vi "Module - RH_JENGENG.vi"() -> ()   [LabVIEW 2019]
uses:
  Control/State - eFGV.ctl
panel:
  out "Site Name":string="RH BELAJA (22.75 kWp)"
  out "STP-03-B-IDC":dbl caption="B.Idc" format="%.1f A"
  out "STP-03-B-VDC":dbl caption="B.Vdc" format="%.0f V"
  out "STP-02-B-IDC":dbl caption="B.Idc" format="%.1f A"
  out "STP-02-B-VDC":dbl caption="B.Vdc" format="%.0f V"
  out "STP-01-B-IDC":dbl caption="B.Idc" format="%.1f A"
  out "STP-01-B-VDC":dbl caption="B.Vdc" format="%.0f V"
  out "BANK-04-STATUS":bool
  out "BANK-03-STATUS":bool
  out "BANK-02-STATUS":bool
  out "BANK-01-STATUS":bool
  out "BANK-04-TEMP":dbl caption="T_bat" format="%#_g °C"
  out "BANK-04-IDC":dbl caption="I_bat" format="%.2f A"
  out "BANK-04-VDC":dbl caption="V_bat" format="%.1f V"
  out "BANK-04-SOC":dbl caption="SOC" format="%#_g %"
  out "BANK-03-TEMP":dbl caption="T_bat" format="%#_g °C"
  out "BANK-03-IDC":dbl caption="I_bat" format="%.2f A"
  out "BANK-03-VDC":dbl caption="V_bat" format="%.1f V"
  out "BANK-03-SOC":dbl caption="SOC" format="%#_g %"
  out "SI-M-02-STATUS":bool
  out "SI-M-02-FREQ":dbl caption="FREQ" format="%.0f Hz"
  out "SI-M-02-L3":dbl caption="L3" format="%.0f V"
  out "SI-M-02-L2":dbl caption="L2" format="%.0f V"
  out "SI-M-02-L1":dbl caption="L1" format="%.0f V"
  out "SI-M-02-PAC":dbl caption="Pac" format="%.0f W"
  out "STP-03-STATUS":bool
  out "STP-03-A-IDC":dbl caption="A.Idc" format="%.1f A"
  out "STP-03-A-VDC":dbl caption="A.Vdc" format="%.0f V"
  out "STP-03-PAC":dbl caption="Pac" format="%#_g W"
  out "PM-01-STATUS":bool
  out "SI-M-01-STATUS":bool
  out "STP-02-STATUS":bool
  out "STP-01-STATUS":bool
  out "BANK-02-TEMP":dbl caption="T_bat" format="%#_g °C"
  out "BANK-02-IDC":dbl caption="I_bat" format="%.2f A"
  out "BANK-02-VDC":dbl caption="V_bat" format="%.1f V"
  out "BANK-02-SOC":dbl caption="SOC" format="%#_g %"
  out "STP-02-A-IDC":dbl caption="A.Idc" format="%.1f A"
  out "STP-02-A-VDC":dbl caption="A.Vdc" format="%.0f V"
  out "STP-02-PAC":dbl caption="Pac" format="%#_g W"
  out "PM-01-FREQ":dbl caption="Freq" format="%.0f Hz"
  out "PM-01-IAC":dbl caption="Iac" format="%.0f A"
  out "PM-01-VAC":dbl caption="Vac" format="%.0f V"
  out "PM-01-PAC":dbl caption="Pac" format="%.0f W"
  out "SI-M-01-FREQ":dbl caption="FREQ" format="%.0f Hz"
  out "SI-M-01-L3":dbl caption="L3" format="%.0f V"
  out "SI-M-01-L2":dbl caption="L2" format="%.0f V"
  out "SI-M-01-L1":dbl caption="L1" format="%.0f V"
  out "SI-M-01-PAC":dbl caption="Pac" format="%.0f W"
  out "BANK-01-TEMP":dbl caption="T_bat" format="%#_g °C"
  out "BANK-01-IDC":dbl caption="I_bat" format="%.2f A"
  out "BANK-01-VDC":dbl caption="V_bat" format="%.1f V"
  out "BANK-01-SOC":dbl caption="SOC" format="%#_g %"
  out "STP-01-A-IDC":dbl caption="A.Idc" format="%.1f A"
  out "STP-01-A-VDC":dbl caption="A.Vdc" format="%.0f V"
  out "STP-01-PAC":dbl caption="Pac" format="%.0f W"
  # "RH JENGENG (30.3 kWp)"
  # "BANK-1"
  # "BANK-2"
  # "BANK-1"
  # "BANK-2"
  # "STP-01"
  # "STP-02"
  # "SI-M-01"
  # "SI-M-02"
  # "STP-03"
  # "PM-01"
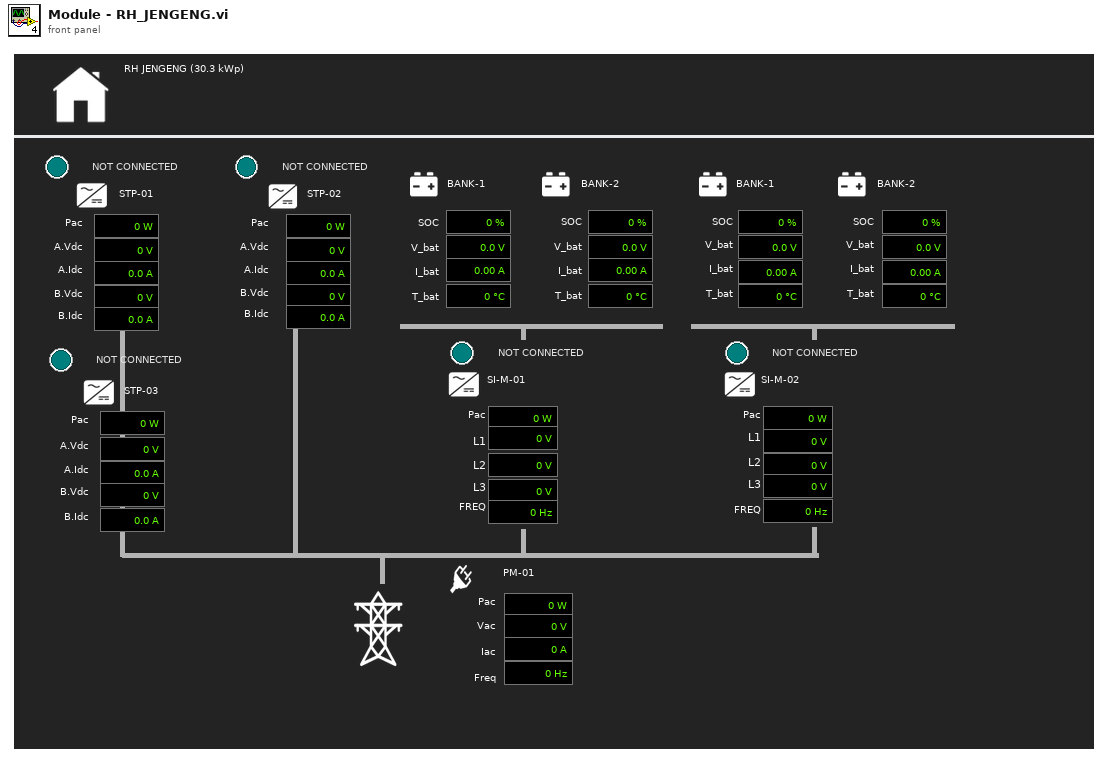
[diagram p1: front panel]
types:
  T1 = typedef "State - eFGV.ctl" = enum16{"Init", "Read", "Write", "Close"}
  T2 = typedef "Device Name.ctl" = enum16{"SB-01", "SB-02", "SB-03", "SB-04", "STP-01", "STP-02", "STP-03", "STP-04", "BANK-01", "BANK-02", "BANK-03", "BANK-04", "SI-M-01", "SI-M-02", "SI-M-03", "SI-M-04", "PM-01", "PM-02", "PM-03", "PM-04"}
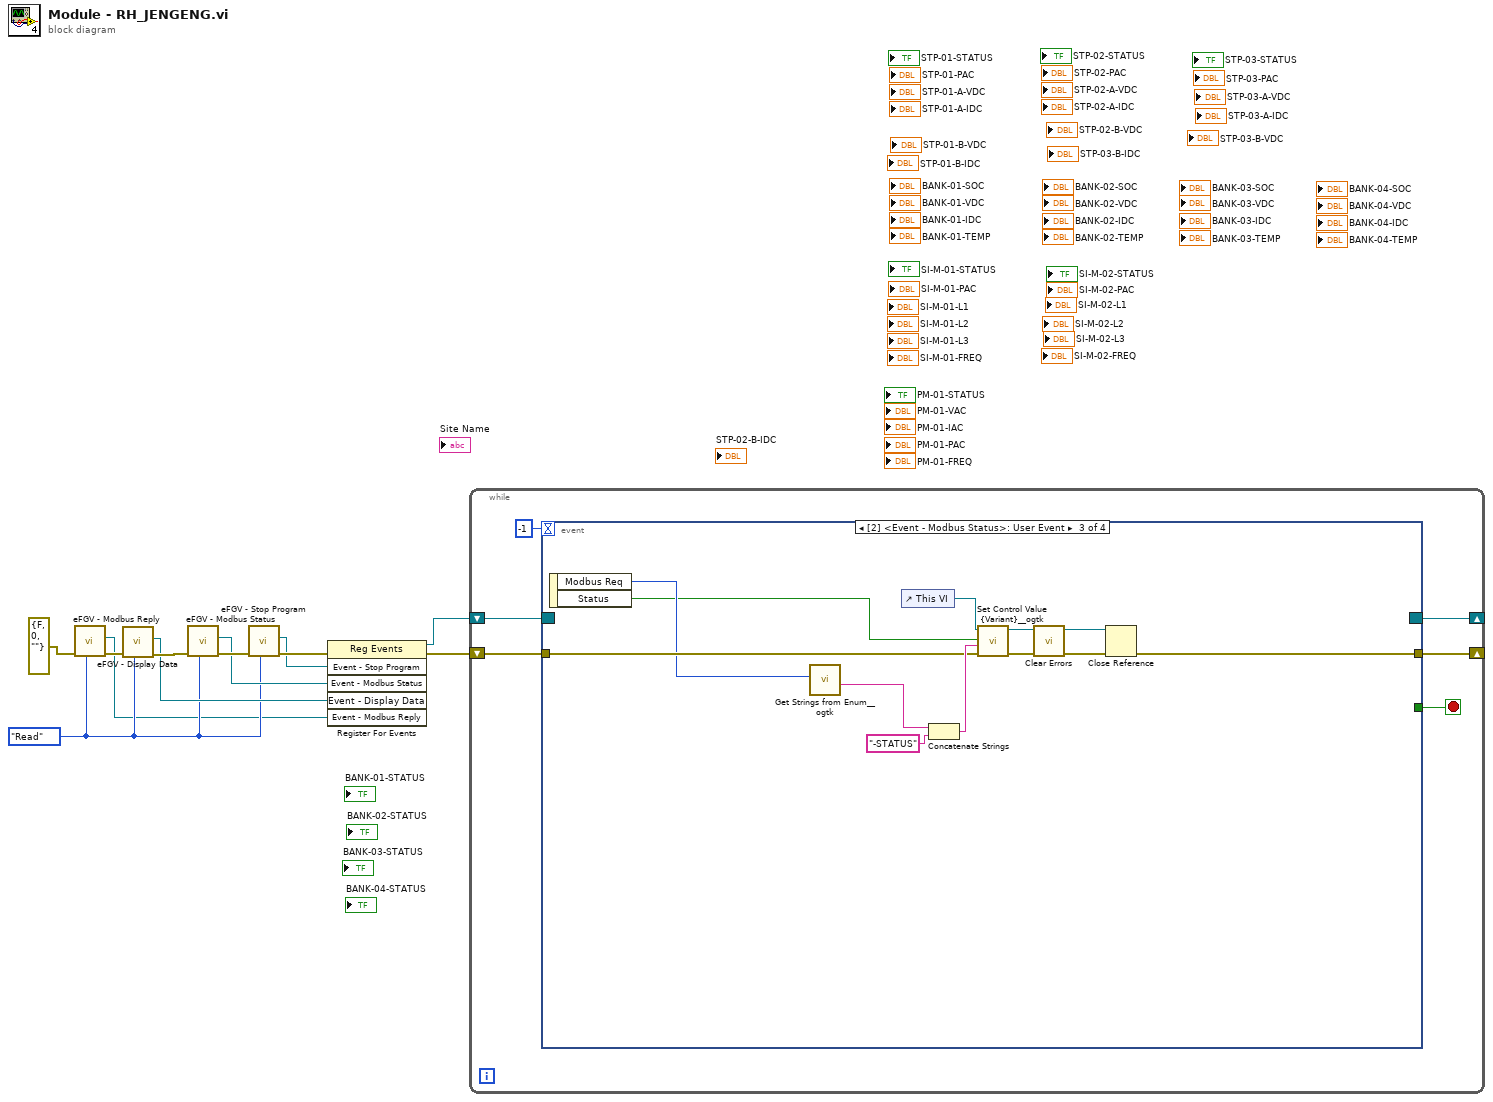
[diagram p0: block diagram]
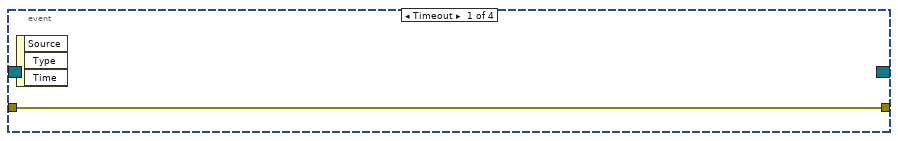
[diagram p2: hidden frame]
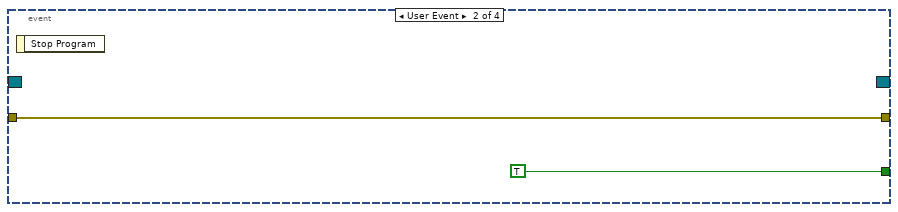
[diagram p3: hidden frame]
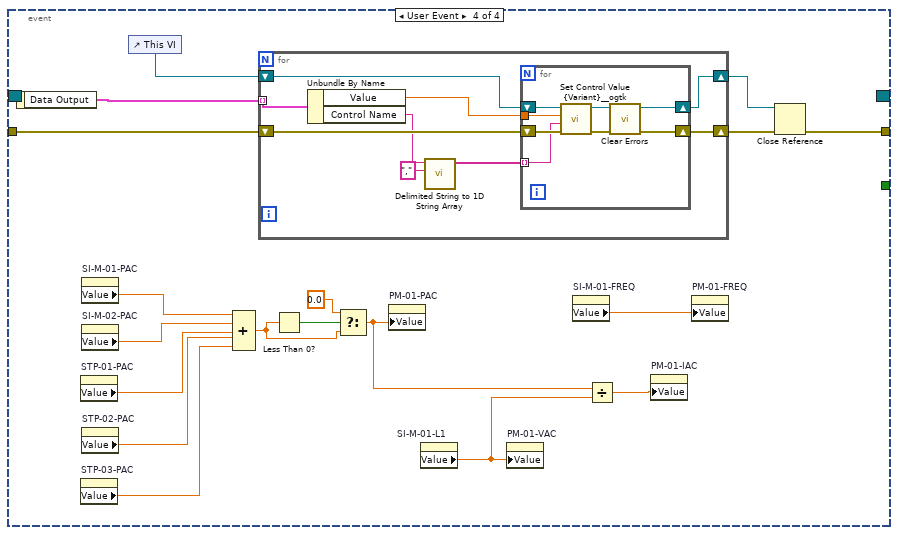
[diagram p4: hidden frame]
diagram:
  w2 = State_-_eFGV."Read" ("State - eFGV")
  n1 = call "eFGV - Modbus Reply.vi"("State - eFGV"=w2, "error in (no error)"=errorcluster {"status"=FALSE, "code"=0, "source"=""}) -> ("error out"=w3:errorcluster, "Event - Modbus Reply"=w1:refnum<user-event>)  [unwired: 8 in]
  n2 = call "eFGV - Display Data.vi"("State - eFGV"=w2, "error in (no error)"=w3) -> ("error out"=w7:errorcluster, "Event - Display Data"=w6:refnum<user-event>)  [unwired: 8 in]
  n3 = call "eFGV - Modbus Status.vi"("State - eFGV"=w2, "error in (no error)"=w7) -> ("error out"=w9:errorcluster, "Event - Modbus Status"=w8:refnum<user-event>)  [unwired: 8 in]
  n4 = call "eFGV - Stop Program.vi"("State - eFGV"=w2, "error in (no error)"=w9) -> ("error out"=w12:errorcluster, "Event - Stop Program"=w11:refnum<user-event>)  [unwired: 8 in]
  n5 = register-events(error in=w12, w11, w8, w6, w1) -> (reference out=w10:refnum<event-registration>, error out=w5:errorcluster)  [unwired: 1 in]
  n6 = while {
    shift-right: [w17] -> _
    shift-left: w10 -> [w18]
    shift-right: [w14] -> _
    shift-left: w5 -> [w13]
    stop <- w16 stop-if-true
    n7 = event shown="[2] <Event - Modbus Status>: User Event" {
      selector: w18 -> [_ _ _ _]
      dyn-events: [_ _ _ _] -> w17
      timeout: -1 -> [_ _ _ _]
      tunnel: w13 -> [w19 w20 w26 w46]
      tunnel: [_ TRUE _ _] -> w16
      tunnel: [w19 w20 w23 w48] -> w14
      event Timeout {
        n8 = event-data() -> ()  [unwired: 1 in, 3 out]
      }
      event User Event {
        n9 = event-data() -> ()  [unwired: 1 in, 1 out]
      }
      event User Event {
        n10 = event-data() -> ("Modbus Req"=w25:T2, "Status"=w24:bool)  [unwired: 1 in]
        n11 = call "Get Strings from Enum__ogtk.vi"("Enum"=w25) -> ("String Value"=w28:string)  [unwired: 7 in, 3 out]
        n12 = control-ref of="This VI"() -> (w32:refnum<vi>)
        n13 = Concatenate Strings(w28, "-STATUS" ("string")) -> (w31:string)
        n14 = call "Set Control Value {Variant}__ogtk.vi"("error in (no error)"=w26, "Control Name (\"\": use variant name)"=w31, "Value"=w24, "VI Refnum"=w32) -> ("error out"=w30:errorcluster, "VI Refnum dup"=w29:refnum<vi>)  [unwired: 6 in]
        n15 = call <vilib>:"Clear Errors.vi"("error in (no error)"=w30) -> ("error out"=w22:errorcluster)  [unwired: 5 in, 1 out]
        n16 = Close Reference(reference=w29, error in (no error)=w22) -> (error out=w23:errorcluster)
      }
      event User Event {
        n17 = event-data() -> ("Data Output"=w47:cluster{"Control Name":string, "Value":dbl}[])  [unwired: 1 in]
        n18 = property on="STP-01-PAC" class="DigNum (strict)"() -> ("Value"=w42:dbl)  [unwired: 2 in, 2 out]
        n19 = property on="STP-03-PAC" class="DigNum (strict)"() -> ("Value"=w34:dbl)  [unwired: 2 in, 2 out]
        n20 = property on="SI-M-01-PAC" class="DigNum (strict)"() -> ("Value"=w44:dbl)  [unwired: 2 in, 2 out]
        n21 = property on="SI-M-02-PAC" class="DigNum (strict)"() -> ("Value"=w43:dbl)  [unwired: 2 in, 2 out]
        n22 = property on="STP-02-PAC" class="DigNum (strict)"() -> ("Value"=w35:dbl)  [unwired: 2 in, 2 out]
        n23 = control-ref of="This VI"() -> (w33:refnum<vi>)
        n24 = Compound Arithmetic op=ADD(w44, w43, w42, w35, w34) -> (w40:dbl)
        n25 = for {
          tunnel: w47 -> [w56] mode=indexing
          shift-right: [w58] -> w50
          shift-left: w46 -> [w59]
          shift-right: [w57] -> w49
          shift-left: w33 -> [w51]
          n26 = Unbundle By Name(w56) -> ("Value"=w55:dbl, "Control Name"=w54:string)
          n27 = call <vilib>:"Delimited String to 1D String Array.vi"("delimiter"=",", "delimited string"=w54) -> ("string array"=w52:string[])  [unwired: 9 in]
          n28 = for {
            tunnel: w55 -> [w62]
            shift-right: [w63] -> w57
            shift-left: w51 -> [w66]
            shift-right: [w60] -> w58
            shift-left: w59 -> [w65]
            tunnel: w52 -> [w61] mode=indexing
            n29 = call "Set Control Value {Variant}__ogtk.vi"("error in (no error)"=w65, "Control Name (\"\": use variant name)"=w61, "Value"=w62, "VI Refnum"=w66) -> ("error out"=w64:errorcluster, "VI Refnum dup"=w63:refnum<vi>)  [unwired: 6 in]
            n30 = call <vilib>:"Clear Errors.vi"("error in (no error)"=w64) -> ("error out"=w60:errorcluster)  [unwired: 5 in, 1 out]
          }
        }
        n31 = Less Than 0?(x=w40) -> (x < 0?=w41:bool)
        n32 = Select(t=0.0, s=w41, f=w40) -> (s? t:f=w37:dbl)
        n33 = property on="PM-01-PAC" class="DigNum (strict)"("Value"=w37) -> ()  [unwired: 2 in, 2 out]
        n34 = property on="SI-M-01-L1" class="DigNum (strict)"() -> ("Value"=w36:dbl)  [unwired: 2 in, 2 out]
        n35 = property on="PM-01-VAC" class="DigNum (strict)"("Value"=w36) -> ()  [unwired: 2 in, 2 out]
        n36 = property on="SI-M-01-FREQ" class="DigNum (strict)"() -> ("Value"=w45:dbl)  [unwired: 2 in, 2 out]
        n37 = Divide(x=w37, y=w36) -> (x/y=w38:dbl)
        n38 = property on="PM-01-IAC" class="DigNum (strict)"("Value"=w38) -> ()  [unwired: 2 in, 2 out]
        n39 = property on="PM-01-FREQ" class="DigNum (strict)"("Value"=w45) -> ()  [unwired: 2 in, 2 out]
        n40 = Close Reference(reference=w49, error in (no error)=w50) -> (error out=w48:errorcluster)
      }
    }
  }
